vi "WaitGenerateExersice.vi"(8 "error in":errorcluster, 10 "VI reference":refnum<vi>, 11 "Notifier in":refnum<notifier>) -> (0 "error out":errorcluster)   [LabVIEW 2014]
uses:
  Ctls/ExerciseMngt.ctl
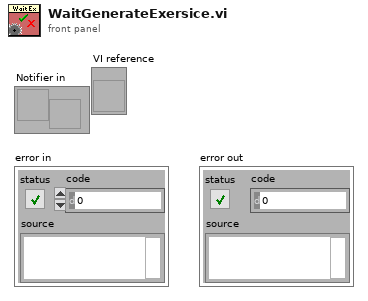
[diagram p1: front panel]
types:
  T1 = typedef "ExerciseMngt.ctl" = enum16{"Timeout", "Generating Exercise", "Exercise Generated"}
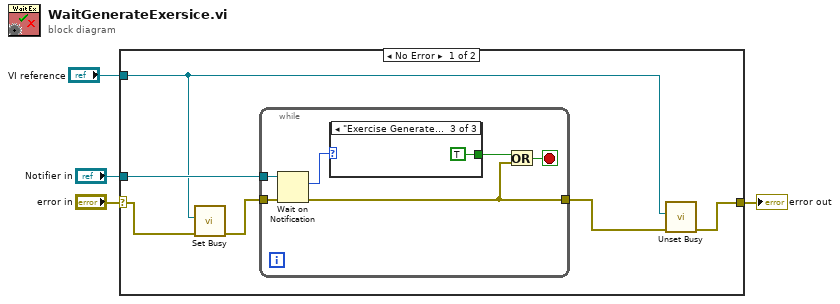
[diagram p0: block diagram]
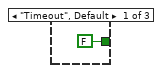
[diagram p2: hidden frame]
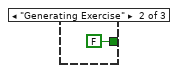
[diagram p3: hidden frame]
diagram:
  n1 = case shown="No Error" "error in" {
    selector: "error in" -> [w9 w20]
    tunnel: [w6 w20] -> w4
    tunnel: "Notifier in" -> [w10 _]
    tunnel: "VI reference" -> [w5 _]
    frame No Error {
      n2 = call <vilib>:"Set Busy.vi"("error in (no error)"=w9, "VI reference (current VI)"=w5) -> ("error out"=w8:errorcluster)  [unwired: 8 in, 1 out]
      n3 = while {
        tunnel: w10 -> [w16]
        tunnel: w8 -> [w14]
        tunnel: [w11] -> w7
        stop <- w13 stop-if-true
        n4 = Wait on Notification(notifier=w16, error in (no error)=w14) -> (notification=w15:T1, error out=w11:errorcluster)  [unwired: 2 in, 2 out]
        n5 = case shown="\"Exercise Generated\"" w15 {
          tunnel: [FALSE FALSE TRUE] -> w12
          frame "Timeout", Default {
          }
          frame "Generating Exercise" {
          }
          frame "Exercise Generated" {
          }
        }
        n6 = Or(x=w12, y=w11) -> (x .or. y?=w13:bool)
      }
      n7 = call <vilib>:"Unset Busy.vi"("error in (no error)"=w7, "VI reference (current VI)"=w5) -> ("error out"=w6:errorcluster)  [unwired: 9 in]
    }
    frame Error {
    }
  }
  "error out" <- w4
